vi "9215_Q.vi"(7 "cmd":enum16{"close", "write", "read", "create"}(ring), 8 "error in":errorcluster, 11 "data":enum16{"stop", "start"}(ring)) -> (0 "error out":errorcluster, 3 "queue out":refnum<queue>)   [LabVIEW 2013]
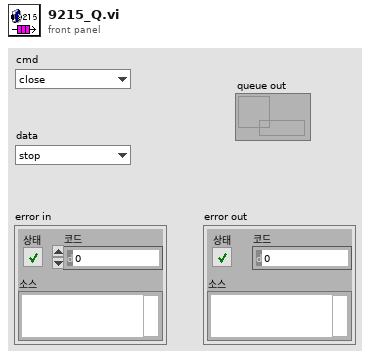
[diagram p1: front panel]
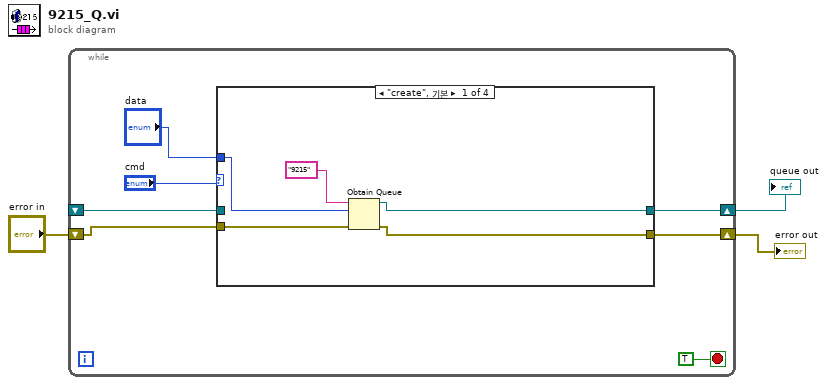
[diagram p0: block diagram]
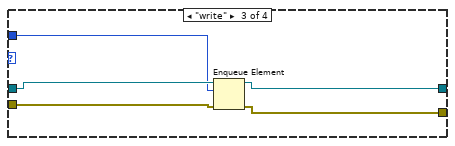
[diagram p3: hidden frame]
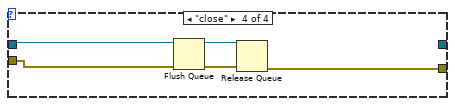
[diagram p4: hidden frame]
diagram:
  n1 = while {
    shift-right: [w6] -> w1
    shift-left: _ -> [w5]
    shift-right: [w7] -> w3
    shift-left: "error in" -> [w8]
    stop <- TRUE stop-if-true
    n2 = case shown="\"create\", 기본" "cmd" {
      tunnel: w8 -> [w15 w17 w22 w23]
      tunnel: [w14 w17 w19 w26] -> w7
      tunnel: [w13 w16 w20 _] -> w6
      tunnel: w5 -> [_ w16 w21 w24]
      tunnel: "data" -> [w11 _ w18 _]
      frame "create", Default {
        n3 = Obtain Queue(name (unnamed)="9215" ("이름(이름없음)"), element data type=w11, error in (no error)=w15) -> (queue out=w13:refnum<queue>, error out=w14:errorcluster)  [unwired: 2 in, 1 out]
      }
      frame "read" {
      }
      frame "write" {
        n4 = Enqueue Element(queue=w21, element=w18, error in (no error)=w22) -> (queue out=w20:refnum<queue>, error out=w19:errorcluster)  [unwired: 1 in, 1 out]
      }
      frame "close" {
        n5 = Flush Queue(queue=w24, error in (no error)=w23) -> (queue out=w25:refnum<queue>, error out=w27:errorcluster)  [unwired: 1 out]
        n6 = Release Queue(queue=w25, error in (no error)=w27) -> (error out=w26:errorcluster)  [unwired: 1 in, 2 out]
      }
    }
  }
  "error out" <- w3
  "queue out" <- w1
